vi "testZTAAC.vi"(8 "error in (no error)":errorcluster) -> (0 "error out":errorcluster)   [LabVIEW 2016]
doc: "Test the ZTAAC class."
uses:
  <vilib>/addons/_JKI Toolkits/Caraya/classes/Test/Test.lvclass
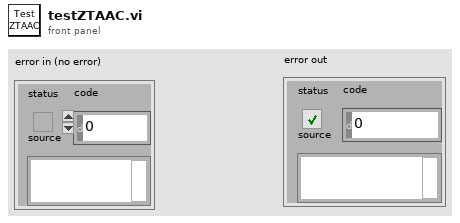
[diagram p1: front panel]
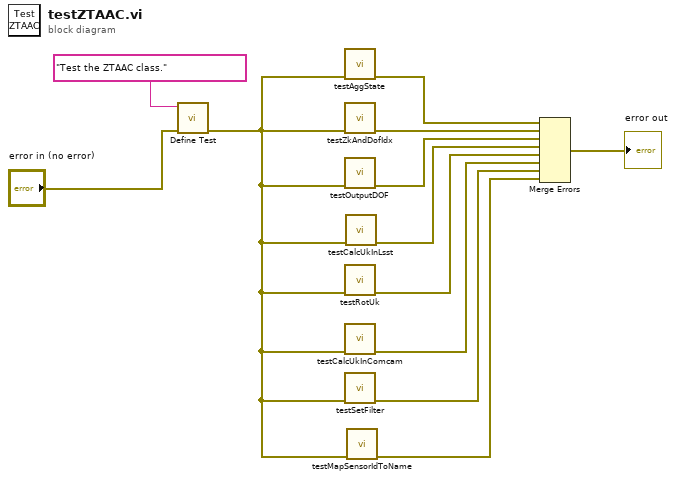
[diagram p0: block diagram]
diagram:
  n1 = call <vilib>:"Define Test.vi"("error in (no error)"="error in (no error)", "Label (VI Title)"="Test the ZTAAC class.") -> ("error out"=w2:errorcluster)  [unwired: 9 in]
  n2 = call "testAggState.vi"("error in (no error)"=w2) -> ("error out"=w11:errorcluster)  [unwired: 10 in]
  n3 = call "testZkAndDofIdx.vi"("error in (no error)"=w2) -> ("error out"=w10:errorcluster)  [unwired: 10 in]
  n4 = call "testOutputDOF.vi"("error in (no error)"=w2) -> ("error out"=w9:errorcluster)  [unwired: 10 in]
  n5 = call "testRotUk.vi"("error in (no error)"=w2) -> ("error out"=w5:errorcluster)  [unwired: 10 in]
  n6 = call "testCalcUkInComcam.vi"("error in (no error)"=w2) -> ("error out"=w4:errorcluster)  [unwired: 10 in]
  n7 = call "testSetFilter.vi"("error in (no error)"=w2) -> ("error out"=w3:errorcluster)  [unwired: 10 in]
  n8 = call "testCalcUkInLsst.vi"("error in (no error)"=w2) -> ("error out"=w6:errorcluster)  [unwired: 10 in]
  n9 = call "testMapSensorIdToName.vi"("error in (no error)"=w2) -> ("error out"=w1:errorcluster)  [unwired: 10 in]
  n10 = Merge Errors(w11, w10, w9, w6, w5, w4, w3, w1) -> (→"error out":errorcluster)
